vi "LDM111 main.vi"() -> ()   [LabVIEW 2012]
uses:
  <vilib>/DAQmx/read.llb/DAQmx Read (Analog 2D DBL NChan NSamp).vi
  <vilib>/DAQmx/write.llb/DAQmx Write (Digital 1D Bool 1Chan 1Samp).vi
  <vilib>/DAQmx/create/channels.llb/DAQmx Create Channel (CO-Pulse Generation-Frequency).vi
  <vilib>/DAQmx/configure/timing.llb/DAQmx Timing (Implicit).vi
  <vilib>/DAQmx/create/channels.llb/DAQmx Create Channel (AI-Voltage-Basic).vi
  <vilib>/DAQmx/configure/timing.llb/DAQmx Timing (Sample Clock).vi
  <vilib>/DAQmx/create/channels.llb/DAQmx Create Channel (DO-Digital Output).vi
  <vilib>/DAQmx/miscellaneous.llb/DAQmx Fill In Error Info.vi
  <resource>/objmgr/daqmx.rc
panel:
  in  "保存间隔时间":u64=1 min=1 step=1
  out "当前湿度":dbl min=0.0 format="%#.2f"
  in  "参数一致":bool
  in  "4-6参数设置":T1={"1-1"={TRUE, "占空比"=enum."100%", "运行时间"=99.0, "电压设置"=0.0}, "1-1 2"={FALSE, "占空比"=enum."0%", "运行时间"=0.0, "电压设置"=0.0}, "1-1 3"={FALSE, "占空比"=enum."0%", "运行时间"=0.0, "电压设置"=0.0}, "1-1 4"={FALSE, "占空比"=enum."0%", "运行时间"=0.0, "电压设置"=0.0}, "1-1 5"={FALSE, "占空比"=enum."0%", "运行时间"=0.0, "电压设置"=0.0}, "1-1 6"={FALSE, "占空比"=enum."0%", "运行时间"=0.0, "电压设置"=0.0}} {"1-1 6"."电压设置" min=0.0 format="%#.2f"; "1-1 6"."运行时间" min=0.0 format="%#.2f"; "1-1 5"."电压设置" min=0.0 format="%#.2f"; "1-1 5"."运行时间" min=0.0 format="%#.2f"; "1-1 4"."电压设置" min=0.0 format="%#.2f"; "1-1 4"."运行时间" min=0.0 format="%#.2f"; "1-1 3"."电压设置" min=0.0 format="%#.2f"; "1-1 3"."运行时间" min=0.0 format="%#.2f"; "1-1 2"."电压设置" min=0.0 format="%#.2f"; "1-1 2"."运行时间" min=0.0 format="%#.2f"; "1-1"."电压设置" min=0.0 format="%#.2f"; "1-1"."运行时间" min=0.0 format="%#.2f"}
  in  "1-3参数设置":T1={"1-1"={TRUE, "占空比"=enum."100%", "运行时间"=99.0, "电压设置"=13.5}, "1-1 2"={FALSE, "占空比"=enum."0%", "运行时间"=0.0, "电压设置"=0.0}, "1-1 3"={FALSE, "占空比"=enum."0%", "运行时间"=0.0, "电压设置"=0.0}, "1-1 4"={FALSE, "占空比"=enum."0%", "运行时间"=0.0, "电压设置"=0.0}, "1-1 5"={FALSE, "占空比"=enum."0%", "运行时间"=0.0, "电压设置"=0.0}, "1-1 6"={FALSE, "占空比"=enum."0%", "运行时间"=0.0, "电压设置"=0.0}} {"1-1 6"."电压设置" min=0.0 format="%#.2f"; "1-1 6"."运行时间" min=0.0 format="%#.2f"; "1-1 5"."电压设置" min=0.0 format="%#.2f"; "1-1 5"."运行时间" min=0.0 format="%#.2f"; "1-1 4"."电压设置" min=0.0 format="%#.2f"; "1-1 4"."运行时间" min=0.0 format="%#.2f"; "1-1 3"."电压设置" min=0.0 format="%#.2f"; "1-1 3"."运行时间" min=0.0 format="%#.2f"; "1-1 2"."电压设置" min=0.0 format="%#.2f"; "1-1 2"."运行时间" min=0.0 format="%#.2f"; "1-1"."电压设置" min=0.0 format="%#.2f"; "1-1"."运行时间" min=0.0 format="%#.2f"}
  in  "剩余时间":dbl min=0.0 format="%#.2f"
  in  "已运行时间":dbl min=0.0 format="%#.2f"
  in  "设定运行时间":dbl=999.0 min=0.0 format="%#.2f"
  in  "停止":bool
  in  "开始":bool
  out "当前温度":dbl min=0.0 format="%#.2f"
  out "工位6":T3={"输入电压"=0.0, "输入电流"=0.0, "输出电压"=0.0, "输出电流"=0.0, "工作效率"=0.0, "占空比"=0.0, "结果"=2.0} {"占空比" format="%#.2g"; "工作效率" format="%#.3f"; "输出电流" format="%#.1f"; "输出电压" format="%#.2f"; "输入电流" format="%#.1f"; "输入电压" format="%#.2f"}
  out "工位5":T3={"输入电压"=0.0, "输入电流"=0.0, "输出电压"=0.0, "输出电流"=0.0, "工作效率"=0.0, "占空比"=0.0, "结果"=2.0} {"占空比" format="%#.2g"; "工作效率" format="%#.3f"; "输出电流" format="%#.1f"; "输出电压" format="%#.2f"; "输入电流" format="%#.1f"; "输入电压" format="%#.2f"}
  out "工位4":T3={"输入电压"=0.0, "输入电流"=0.0, "输出电压"=0.0, "输出电流"=0.0, "工作效率"=0.0, "占空比"=0.0, "结果"=2.0} {"占空比" format="%#.2g"; "工作效率" format="%#.3f"; "输出电流" format="%#.1f"; "输出电压" format="%#.2f"; "输入电流" format="%#.1f"; "输入电压" format="%#.2f"}
  out "工位3":T3={"输入电压"=0.0, "输入电流"=0.0, "输出电压"=0.0, "输出电流"=0.0, "工作效率"=0.0, "占空比"=0.0, "结果"=2.0} {"占空比" format="%#.2g"; "工作效率" format="%#.3f"; "输出电流" format="%#.1f"; "输出电压" format="%#.2f"; "输入电流" format="%#.1f"; "输入电压" format="%#.2f"}
  out "工位2":T3={"输入电压"=0.0, "输入电流"=0.0, "输出电压"=0.0, "输出电流"=0.0, "工作效率"=0.0, "占空比"=0.0, "结果"=2.0} {"占空比" format="%#.2g"; "工作效率" format="%#.3f"; "输出电流" format="%#.1f"; "输出电压" format="%#.2f"; "输入电流" format="%#.1f"; "输入电压" format="%#.2f"}
  out "工位1":T3={"输入电压"=0.0, "输入电流"=0.0, "输出电压"=0.0, "输出电流"=0.0, "工作效率"=0.0, "占空比"=0.0, "结果"=2.0} {"占空比" format="%#.2g"; "工作效率" format="%#.3f"; "输出电流" format="%#.1f"; "输出电压" format="%#.2f"; "输入电流" format="%#.1f"; "输入电压" format="%#.2f"}
  # "LDM111"
  # "V"
  # "MA"
  # "V"
  # "MA"
  # "C"
  # "min"
  # "%"
  # "%"
  # "%"
  # "%"
  # "%"
  # "%"
  # "min"
  # "min"
  # "参数一致?"
  # "s"
  # "V"
  # "启用"
  # "min"
  # "V"
  # "启用"
  # "min"
  # "V"
  # "启用"
  # "min"
  # "启用"
  # "min"
  # "V"
  # "V"
  # "启用"
  # "min"
  # "启用"
  # "min"
  # "V"
  # "启用"
  # "V"
  # "min"
  # "启用"
  # "V"
  # "min"
  # "启用"
  # "V"
  # "min"
  # "启用"
  # "V"
  # "min"
  # "启用"
  # "V"
  # "min"
  # "启用"
  # "V"
  # "min"
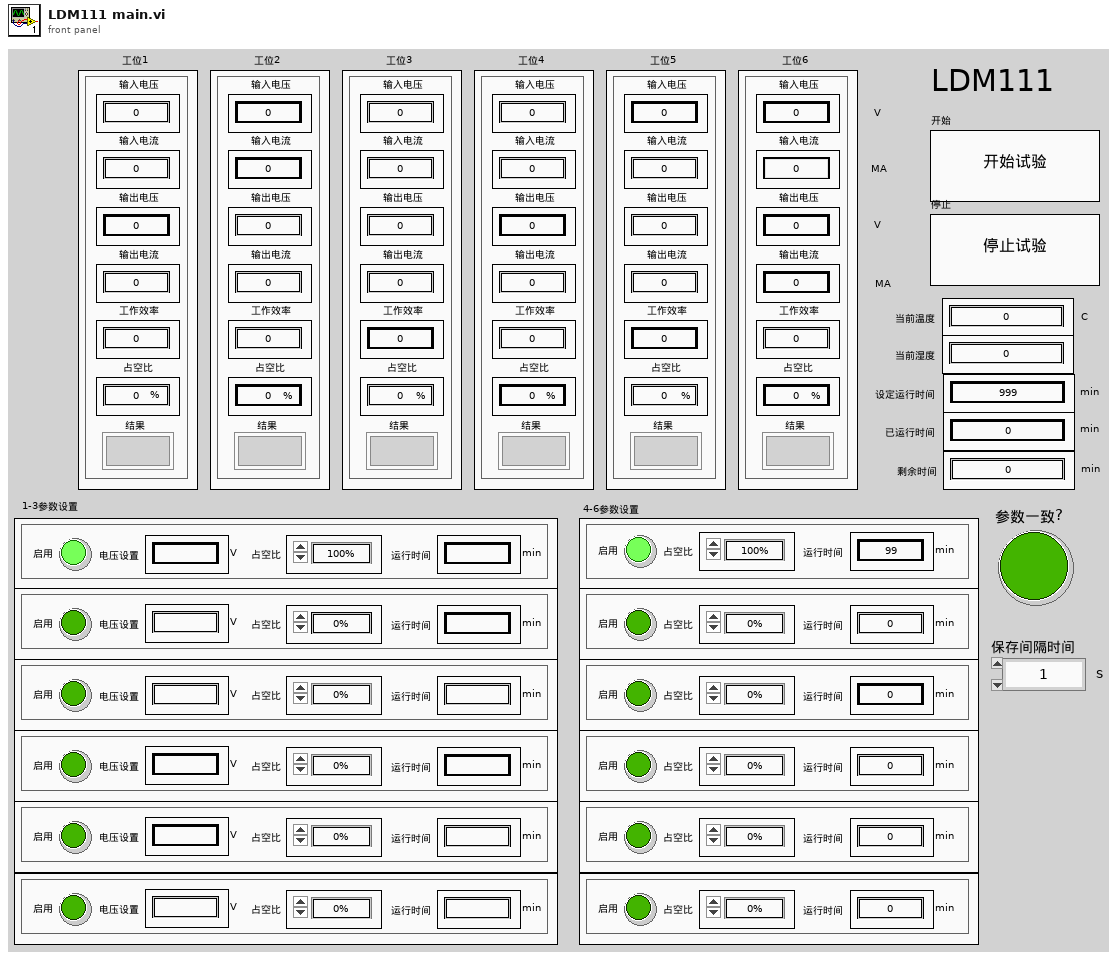
[diagram p1: front panel]
types:
  T1 = cluster{"1-1":cluster{bool, "占空比":enum16{"0%", "28%", "100%"}, "运行时间":dbl, "电压设置":dbl}, "1-1 2":cluster{bool, "占空比":enum16{"0%", "28%", "100%"}, "运行时间":dbl, "电压设置":dbl}, "1-1 3":cluster{bool, "占空比":enum16{"0%", "28%", "100%"}, "运行时间":dbl, "电压设置":dbl}, "1-1 4":cluster{bool, "占空比":enum16{"0%", "28%", "100%"}, "运行时间":dbl, "电压设置":dbl}, "1-1 5":cluster{bool, "占空比":enum16{"0%", "28%", "100%"}, "运行时间":dbl, "电压设置":dbl}, "1-1 6":cluster{bool, "占空比":enum16{"0%", "28%", "100%"}, "运行时间":dbl, "电压设置":dbl}}
  T2 = typedef "结果状态显示.ctl" = dbl
  T3 = cluster{"输入电压":dbl, "输入电流":dbl, "输出电压":dbl, "输出电流":dbl, "工作效率":dbl, "占空比":dbl, "结果":T2}
  T4 = typedef "控件 1.ctl" = enum16{"初始化", "空闲", "开始", "计时", "完成", "退出"}
  T5 = typedef "控件 3.ctl" = enum16{"初始化", "读取", "写入", "退出"}
  T6 = typedef "控件 2.ctl" = enum16{"创建事件", "产生事件", "销毁事件"}
  T7 = typedef "控件 4.ctl" = cluster{"工位1":refnum<vi>, "1-3参数设置":refnum<vi>, "总时间":u32, "NG？":bool, "循环次数":i32, "步骤次数":i32, "单个时间":u32, "完成?":bool, "路径":path, "1":i32, "2":i32, "3":i32, "4":i32, "AI":i32, "范围":i32, "保存间隔时间":u64}
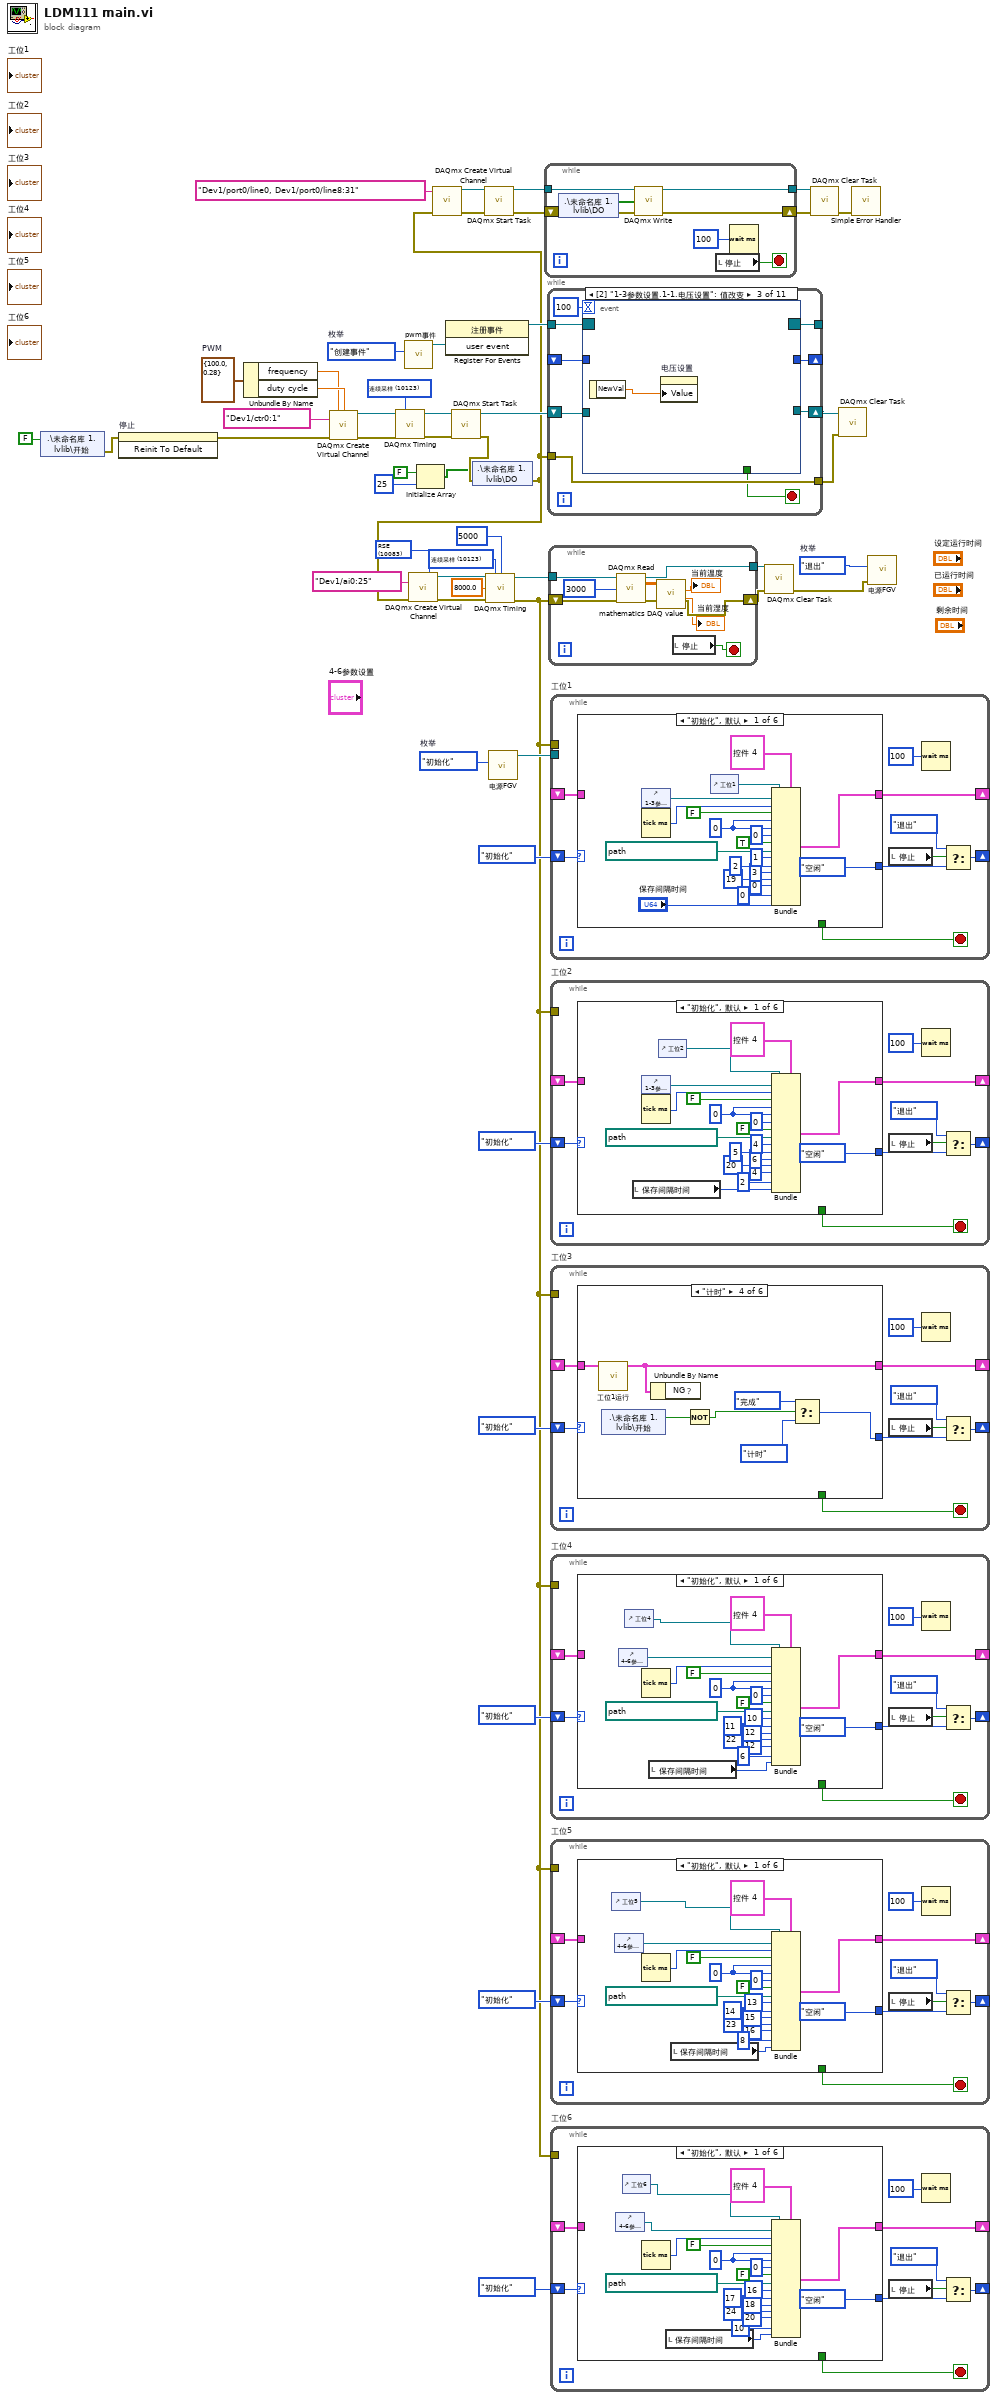
[diagram p0: block diagram]
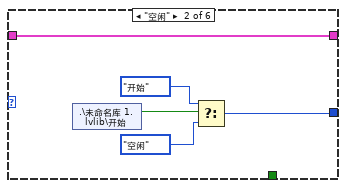
[diagram p2: hidden frame]
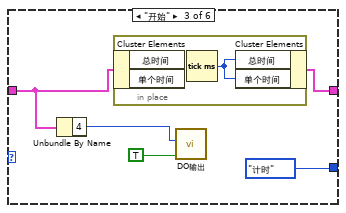
[diagram p3: hidden frame]
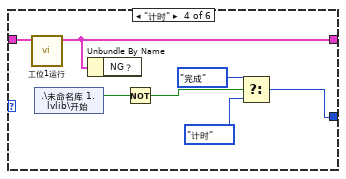
[diagram p4: hidden frame]
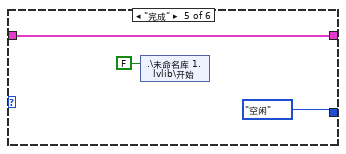
[diagram p5: hidden frame]
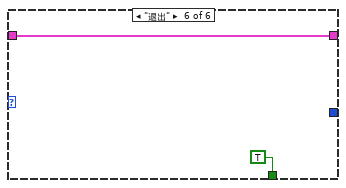
[diagram p6: hidden frame]
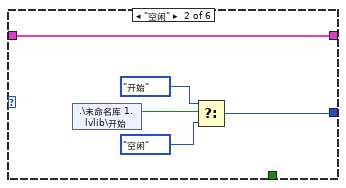
[diagram p7: hidden frame]
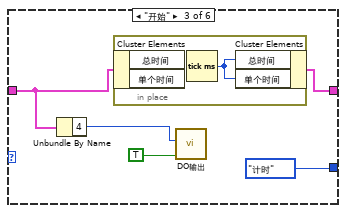
[diagram p8: hidden frame]
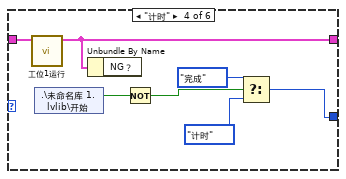
[diagram p9: hidden frame]
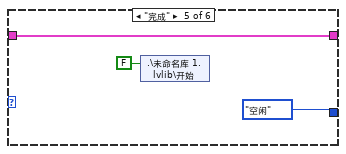
[diagram p10: hidden frame]
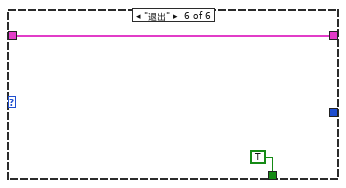
[diagram p11: hidden frame]
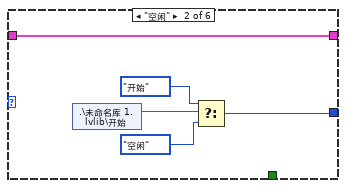
[diagram p12: hidden frame]
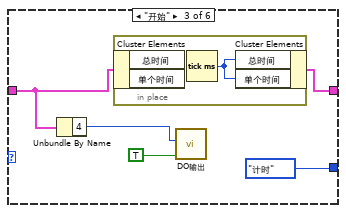
[diagram p13: hidden frame]
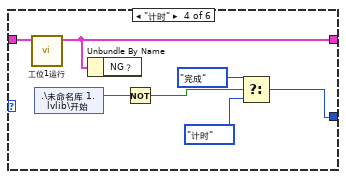
[diagram p14: hidden frame]
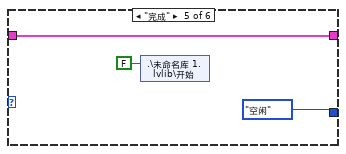
[diagram p15: hidden frame]
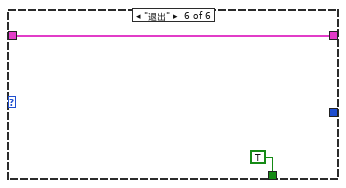
[diagram p16: hidden frame]
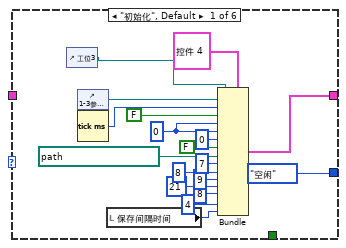
[diagram p17: hidden frame]
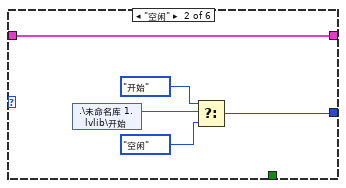
[diagram p18: hidden frame]
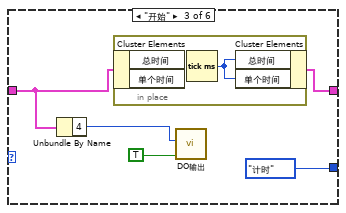
[diagram p19: hidden frame]
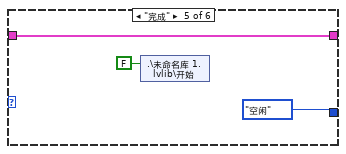
[diagram p20: hidden frame]
diagram:
  w8 = 控件_3."退出"  # 枚举
  w10 = 控件_3."初始化"  # 枚举
  w20 = 10083 items=["默认"=-1, "RSE"=10083, "NRSE"=10078, "差分"=10106, "伪差分"=12529] ("input terminal configuration")
  w22 = 10123 items=["有限采样"=10178, "连续采样"=10123, "硬件定时单点"=12522] ("sample mode")
  w34 = 10123 items=["有限采样"=10178, "连续采样"=10123, "硬件定时单点"=12522] ("sample mode")
  w37 = cluster{"frequency":dbl, "duty cycle":dbl} {"frequency"=100.0, "duty cycle"=0.28}  # PWM
  w44 = 控件_2."创建事件"  # 枚举
  n1 = shared-variable ".\\未命名库 1.lvlib\\开始"(FALSE ("开始")) -> (error out=w11:errorcluster)  [unwired: 1 in]
  n2 = invoke on="停止" class="Bool (严格)" method="Reinit To Default"(error in=w11) -> (error out=w26:errorcluster)  [unwired: 2 in, 2 out]
  n3 = Unbundle By Name(w37) -> ("frequency"=w39:dbl, "duty cycle"=w40:dbl)
  n4 = call-poly <vilib>:"DAQmx Create Virtual Channel.vi"("frequency"=w39, "duty cycle"=w40, "counter"=tag "Dev1/ctr0:1", "error in"=w26) -> ("task out"=w36:refnum<k21>, "error out"=w35:errorcluster)  [unwired: 10 in]
  n5 = call-poly <vilib>:"DAQmx Timing.vi"("task/channels in"=w36, "sample mode"=w34, "error in"=w35) -> ("task out"=w33:refnum<k21>, "error out"=w32:errorcluster)  [unwired: 11 in]
  n6 = call "pwm事件.vi"("枚举"=w44) -> ("user event"=w43:refnum<user-event>)  [unwired: 9 in, 1 out]
  n7 = Initialize Array(FALSE, 25 ("维数大小")) -> (w28:bool[])
  n8 = register-events(w43) -> (reference out=w42:refnum<event-registration>)  [unwired: 2 in, 1 out]
  n9 = call <vilib>:"DAQmx Start Task.vi"("task/channels in"=w33, "error in"=w32) -> ("task out"=w38:refnum<k21>, "error out"=w30:errorcluster)  [unwired: 12 in]
  n10 = shared-variable ".\\未命名库 1.lvlib\\DO"(w28, error in=w30) -> (error out=w17:errorcluster)
  n11 = call-poly <vilib>:"DAQmx Create Virtual Channel.vi"("input terminal configuration"=w20, "physical channels"=tag "Dev1/ai0:25", "error in"=w17) -> ("task out"=w25:refnum<k21>, "error out"=w24:errorcluster)  [unwired: 11 in]
  n12 = call-poly <vilib>:"DAQmx Create Virtual Channel.vi"("lines"=tag "Dev1/port0/line0, Dev1/port0/line8:31" ("Line(s)"), "error in"=w17) -> ("task out"=w45:refnum<k21>, "error out"=w46:errorcluster)  [unwired: 12 in]
  n13 = call <vilib>:"DAQmx Start Task.vi"("task/channels in"=w45, "error in"=w46) -> ("task out"=w52:refnum<k21>, "error out"=w51:errorcluster)  [unwired: 12 in]
  n14 = call-poly <vilib>:"DAQmx Timing.vi"("task/channels in"=w25, "sample mode"=w22, "samples per channel"=5000, "rate"=8000.0, "error in"=w24) -> ("task out"=w18:refnum<k21>, "error out"=w1:errorcluster)  [unwired: 9 in]
  n15 = call "电源FGV.vi"("枚举"=w10) -> ("VISA资源名称输出"=w9:refnum<visa-resource-name>)  [unwired: 9 in, 1 out]
  n16 = while {
    tunnel: w52 -> [w60]
    tunnel: [w59] -> w50
    shift-right: [w58] -> w49
    shift-left: w51 -> [w55]
    stop <- w53 stop-if-true
    n17 = shared-variable ".\\未命名库 1.lvlib\\DO"(error in=w55) -> (w56:bool[], error out=w54:errorcluster)
    n18 = call-poly <vilib>:"DAQmx Write.vi"("task/channels in"=w60, "data"=w56, "error in"=w54) -> ("task out"=w59:refnum<k21>, "error out"=w58:errorcluster)  [unwired: 10 in, 1 out]
    n19 = local read "停止"() -> (w53:bool)
    n20 = Wait (ms)(milliseconds to wait=u32 100 ("Loop Time (ms)")) -> ()  [unwired: 1 out]
  }
  n21 = while {
    tunnel: w42 -> [w69]
    tunnel: w17 -> [w64]
    tunnel: [w67] -> _
    shift-right: [w65] -> w41
    shift-left: w38 -> [w66]
    tunnel: [w64] -> w14
    shift-right: [w62] -> _
    shift-left: _ -> [w61]
    stop <- w63 stop-if-true
    n22 = event shown="[2] \"1-3参数设置.1-1.电压设置\": 值改变" {
      selector: w69 -> [_ _ _ _ _ _ _ _ _ _ _]
      dyn-events: [_ _ _ _ _ _ _ _ _ _ _] -> w67
      timeout: 100 -> [_ _ _ _ _ _ _ _ _ _ _]
      tunnel: w66 -> [w74 _ _ _ _ _ _ _ w84 _ _]
      tunnel: [w74 _ _ _ _ _ _ _ w83 _ _] -> w65
      tunnel: [_ _ _ _ _ _ _ _ _ _ TRUE ("开始")] -> w63
      tunnel: [w70 _ _ _ _ _ _ _ w82 w87 w92] -> w62
      tunnel: w61 -> [w70 _ _ _ _ _ _ _ w82 _ w92]
      event Timeout {
        n23 = event-data() -> ()  [unwired: 1 in, 2 out]
        n24 = control-ref of="剩余时间"() -> (w73:refnum<vi>)
        n25 = control-ref of="已运行时间"() -> (w72:refnum<vi>)
        n26 = control-ref of="设定运行时间"() -> (w71:refnum<vi>)
        n27 = call "总时间.vi"("已运行时间 2"=w72, "剩余时间 2"=w73, "设定运行时间 2"=w71, "millisecond timer value"=w70) -> ()  [unwired: 8 in]
      }
      event "参数一致": Value Change {
        n28 = event-data() -> ()  [unwired: 1 in, 5 out]
        n29 = local write "4-6参数设置"("1-3参数设置") -> ()
      }
      event "1-3参数设置.1-1.电压设置": Value Change {
        n30 = event-data() -> ("NewVal"=w76:dbl)  [unwired: 1 in]
        n31 = property on="电压设置" class="DigNum (严格)"("Value"=w76) -> ()  [unwired: 2 in, 2 out]
      }
      event "1-3参数设置.1-1 2.电压设置": Value Change {
        n32 = event-data() -> ("NewVal"=w77:dbl)  [unwired: 1 in]
        n33 = property on="电压设置" class="DigNum (严格)"("Value"=w77) -> ()  [unwired: 2 in, 2 out]
      }
      event "1-3参数设置.1-1 3.电压设置": Value Change {
        n34 = event-data() -> ("NewVal"=w78:dbl)  [unwired: 1 in]
        n35 = property on="电压设置" class="DigNum (严格)"("Value"=w78) -> ()  [unwired: 2 in, 2 out]
      }
      event "1-3参数设置.1-1 4.电压设置": Value Change {
        n36 = event-data() -> ("NewVal"=w79:dbl)  [unwired: 1 in]
        n37 = property on="电压设置" class="DigNum (严格)"("Value"=w79) -> ()  [unwired: 2 in, 2 out]
      }
      event "1-3参数设置.1-1 5.电压设置": Value Change {
        n38 = event-data() -> ("NewVal"=w80:dbl)  [unwired: 1 in]
        n39 = property on="电压设置" class="DigNum (严格)"("Value"=w80) -> ()  [unwired: 2 in, 2 out]
      }
      event "1-3参数设置.1-1 6.电压设置": Value Change {
        n40 = event-data() -> ("NewVal"=w81:dbl)  [unwired: 1 in]
        n41 = property on="电压设置" class="DigNum (严格)"("Value"=w81) -> ()  [unwired: 2 in, 2 out]
      }
      event User Event {
        n42 = event-data() -> ("frequency"=w86:dbl, "duty cycle"=w85:dbl)  [unwired: 1 in]
        n43 = property class="DAQmx通道"(reference=w84, "CO.Pulse.DutyCyc"=w85, "CO.Pulse.Freq"=w86) -> (reference out=w83:refnum<k21>)  [unwired: 1 in, 1 out]
      }
      event "开始": Value Change {
        n44 = event-data() -> ("NewVal"=w88:bool)  [unwired: 1 in, 1 out]
        n45 = shared-variable ".\\未命名库 1.lvlib\\开始"(w88) -> ()  [unwired: 1 in, 1 out]
        n46 = Tick Count (ms)() -> (millisecond timer value=w87:u32)
      }
      event "停止": Value Change {
        n47 = event-data() -> ()  [unwired: 1 in, 1 out]
        n48 = Initialize Array(FALSE, 25 ("维数大小")) -> (w89:bool[])
        n49 = shared-variable ".\\未命名库 1.lvlib\\DO"(w89) -> ()  [unwired: 1 in, 1 out]
        n50 = shared-variable ".\\未命名库 1.lvlib\\开始"(FALSE ("开始")) -> ()  [unwired: 1 in, 1 out]
      }
    }
  }
  n51 = while {
    tunnel: w18 -> [w102]
    shift-right: [w98] -> w15
    shift-left: w1 -> [w101]
    tunnel: [w100] -> w16
    stop <- w97 stop-if-true
    n52 = call-poly <vilib>:"DAQmx Read.vi"("task/channels in"=w102, "number of samples per channel"=3000, "error in"=w101) -> ("task out"=w100:refnum<k21>, "data"=w99:dbl[][], "error out"=w98:errorcluster)  [unwired: 10 in]
    n53 = call "mathematics DAQ value.vi"("Array"=w99) -> ("湿度?"=→"当前湿度":dbl, "温度?"=→"当前温度":dbl)  [unwired: 4 in, 1 out]
    n54 = local read "停止"() -> (w97:bool)
  }
  n55 = while "工位1" {
    shift-right: [w109] -> _
    shift-left: 控件_1."初始化" ("枚举") -> [w112]
    shift-right: [w108] -> _
    shift-left: _ -> [w107]
    tunnel: w1 -> [_]
    tunnel: w9 -> [_]
    stop <- w105 stop-if-true
    n56 = case shown="\"初始化\", 默认" w112 {
      tunnel: [w128 w131 w139 w147 w151 w153] -> w108
      tunnel: w107 -> [_ w131 w137 w148 w151 w153]
      tunnel: [控件_1."空闲" ("枚举") w132 控件_1."计时" ("枚举") w144 控件_1."空闲" ("枚举") _] -> w106
      tunnel: [_ _ _ _ _ TRUE] -> w105
      frame "初始化", Default {
        w125 = 0 ("步骤次数")
        n57 = control-ref of="1-3参数设置"() -> (w129:refnum<vi>)
        n58 = Tick Count (ms)() -> (millisecond timer value=w127:u32)
        n59 = control-ref of="工位1"() -> (w130:refnum<vi>)
        n60 = Bundle(cluster=T7 {"工位1"=refnum, "1-3参数设置"=refnum, "总时间"=0, "NG？"=FALSE, "循环次数"=0, "步骤次数"=0, "单个时间"=0, "完成?"=FALSE, "路径"=path "e:/LDM数据/工位一", "1"=19, "2"=19, "3"=19, "4"=19, "AI"=24, "范围"=24, "保存间隔时间"=0} ("簇 2"), "工位1"=w130, "1-3参数设置"=w129, "总时间"=w127, "NG？"=FALSE, "循环次数"=w125, "步骤次数"=w125, "单个时间"=u32 0, "完成?"=TRUE, "路径"=path "e:/LDM数据/工位一", "1"=1, "2"=2 ("1"), "3"=3 ("1"), "4"=19 ("1"), "AI"=0 ("1"), "范围"=0 ("1"), "保存间隔时间"="保存间隔时间") -> (w128:T7)
      }
      frame "空闲" {
        n61 = shared-variable ".\\未命名库 1.lvlib\\开始"() -> (w135:bool)  [unwired: 1 in, 1 out]
        n62 = Select(t=控件_1."开始" ("枚举"), s=w135, f=控件_1."空闲" ("枚举")) -> (s? t:f=w132:T4)
      }
      frame "开始" {
        n63 = Unbundle By Name(w137) -> ("4"=w136:i32)
        n64 = in-place {
          n65 = in-place-cluster #1(w137) -> ()  [unwired: 2 out]
          n66 = Tick Count (ms)() -> (millisecond timer value=w141:u32)
          n67 = in-place-cluster #1("总时间"=w141, "单个时间"=w141) -> (w139:T7)
        }
        n68 = call "DO输出.vi"("TF"=TRUE, "序号"=w136) -> ()  [unwired: 9 in, 1 out]
      }
      frame "计时" {
        n69 = call "工位1运行.vi"("簇"=w148) -> ("簇 2"=w147:T7)  [unwired: 10 in]
        n70 = shared-variable ".\\未命名库 1.lvlib\\开始"() -> (w143:bool)  [unwired: 1 in, 1 out]
        n71 = Unbundle By Name(w147) -> ()  [unwired: 1 out]
        n72 = Not(x=w143) -> (.not. x?=w142:bool)
        n73 = Select(t=控件_1."完成" ("枚举"), s=w142, f=控件_1."计时" ("枚举")) -> (s? t:f=w144:T4)
      }
      frame "完成" {
        n74 = shared-variable ".\\未命名库 1.lvlib\\开始"(FALSE ("开始")) -> ()  [unwired: 1 in, 1 out]
      }
      frame "退出" {
      }
    }
    n75 = local read "停止"() -> (w111:bool)
    n76 = Wait (ms)(milliseconds to wait=u32 100 ("等待时间（毫秒）")) -> ()  [unwired: 1 out]
    n77 = Select(t=控件_1."退出" ("枚举"), s=w111, f=w106) -> (s? t:f=w109:T4)
  }
  n78 = while "工位2" {
    shift-right: [w159] -> _
    shift-left: 控件_1."初始化" ("枚举") -> [w162]
    shift-right: [w158] -> _
    shift-left: _ -> [w157]
    tunnel: w1 -> [_]
    stop <- w155 stop-if-true
    n79 = case shown="\"初始化\", 默认" w162 {
      tunnel: [w179 w181 w189 w197 w201 w203] -> w158
      tunnel: w157 -> [_ w181 w187 w198 w201 w203]
      tunnel: [控件_1."空闲" ("枚举") w182 控件_1."计时" ("枚举") w194 控件_1."空闲" ("枚举") _] -> w156
      tunnel: [_ _ _ _ _ TRUE] -> w155
      frame "初始化", Default {
        w176 = 0 ("步骤次数")
        n80 = local read "保存间隔时间"() -> (w163:u64)
        n81 = control-ref of="1-3参数设置"() -> (w180:refnum<vi>)
        n82 = Tick Count (ms)() -> (millisecond timer value=w178:u32)
        n83 = control-ref of="工位2"() -> (w165:refnum<vi>)
        n84 = Bundle(cluster=T7 {"工位1"=refnum, "1-3参数设置"=refnum, "总时间"=0, "NG？"=FALSE, "循环次数"=0, "步骤次数"=0, "单个时间"=0, "完成?"=FALSE, "路径"=path "e:/LDM数据/工位一", "1"=19, "2"=19, "3"=19, "4"=19, "AI"=24, "范围"=24, "保存间隔时间"=0} ("簇 2"), "工位1"=w165, "1-3参数设置"=w180, "总时间"=w178, "NG？"=FALSE, "循环次数"=w176, "步骤次数"=w176, "单个时间"=u32 0, "完成?"=FALSE, "路径"=path "e:/LDM数据/工位二", "1"=4, "2"=5 ("1"), "3"=6 ("1"), "4"=20 ("1"), "AI"=4 ("1"), "范围"=2 ("1"), "保存间隔时间"=w163) -> (w179:T7)
      }
      frame "空闲" {
        n85 = shared-variable ".\\未命名库 1.lvlib\\开始"() -> (w185:bool)  [unwired: 1 in, 1 out]
        n86 = Select(t=控件_1."开始" ("枚举"), s=w185, f=控件_1."空闲" ("枚举")) -> (s? t:f=w182:T4)
      }
      frame "开始" {
        n87 = Unbundle By Name(w187) -> ("4"=w186:i32)
        n88 = in-place {
          n89 = in-place-cluster #2(w187) -> ()  [unwired: 2 out]
          n90 = Tick Count (ms)() -> (millisecond timer value=w191:u32)
          n91 = in-place-cluster #2("总时间"=w191, "单个时间"=w191) -> (w189:T7)
        }
        n92 = call "DO输出.vi"("TF"=TRUE, "序号"=w186) -> ()  [unwired: 9 in, 1 out]
      }
      frame "计时" {
        n93 = call "工位1运行.vi"("簇"=w198) -> ("簇 2"=w197:T7)  [unwired: 10 in]
        n94 = shared-variable ".\\未命名库 1.lvlib\\开始"() -> (w193:bool)  [unwired: 1 in, 1 out]
        n95 = Unbundle By Name(w197) -> ()  [unwired: 1 out]
        n96 = Not(x=w193) -> (.not. x?=w192:bool)
        n97 = Select(t=控件_1."完成" ("枚举"), s=w192, f=控件_1."计时" ("枚举")) -> (s? t:f=w194:T4)
      }
      frame "完成" {
        n98 = shared-variable ".\\未命名库 1.lvlib\\开始"(FALSE ("开始")) -> ()  [unwired: 1 in, 1 out]
      }
      frame "退出" {
      }
    }
    n99 = local read "停止"() -> (w161:bool)
    n100 = Wait (ms)(milliseconds to wait=u32 100 ("等待时间（毫秒）")) -> ()  [unwired: 1 out]
    n101 = Select(t=控件_1."退出" ("枚举"), s=w161, f=w156) -> (s? t:f=w159:T4)
  }
  n102 = while "工位3" {
    shift-right: [w209] -> _
    shift-left: 控件_1."初始化" ("枚举") -> [w212]
    shift-right: [w208] -> _
    shift-left: _ -> [w207]
    tunnel: w1 -> [_]
    stop <- w205 stop-if-true
    n103 = case shown="\"计时\"" w212 {
      tunnel: [w229 w231 w239 w247 w251 w253] -> w208
      tunnel: w207 -> [_ w231 w237 w248 w251 w253]
      tunnel: [控件_1."空闲" ("枚举") w232 控件_1."计时" ("枚举") w244 控件_1."空闲" ("枚举") _] -> w206
      tunnel: [_ _ _ _ _ TRUE] -> w205
      frame "初始化", Default {
        w226 = 0 ("步骤次数")
        n104 = control-ref of="工位3"() -> (w214:refnum<vi>)
        n105 = control-ref of="1-3参数设置"() -> (w230:refnum<vi>)
        n106 = Tick Count (ms)() -> (millisecond timer value=w228:u32)
        n107 = local read "保存间隔时间"() -> (w213:u64)
        n108 = Bundle(cluster=T7 {"工位1"=refnum, "1-3参数设置"=refnum, "总时间"=0, "NG？"=FALSE, "循环次数"=0, "步骤次数"=0, "单个时间"=0, "完成?"=FALSE, "路径"=path "e:/LDM数据/工位一", "1"=19, "2"=19, "3"=19, "4"=19, "AI"=24, "范围"=24, "保存间隔时间"=0} ("簇 2"), "工位1"=w214, "1-3参数设置"=w230, "总时间"=w228, "NG？"=FALSE, "循环次数"=w226, "步骤次数"=w226, "单个时间"=u32 0, "完成?"=FALSE, "路径"=path "e:/LDM数据/工位三", "1"=7, "2"=8 ("1"), "3"=9 ("1"), "4"=21 ("1"), "AI"=8 ("1"), "范围"=4 ("1"), "保存间隔时间"=w213) -> (w229:T7)
      }
      frame "空闲" {
        n109 = shared-variable ".\\未命名库 1.lvlib\\开始"() -> (w235:bool)  [unwired: 1 in, 1 out]
        n110 = Select(t=控件_1."开始" ("枚举"), s=w235, f=控件_1."空闲" ("枚举")) -> (s? t:f=w232:T4)
      }
      frame "开始" {
        n111 = Unbundle By Name(w237) -> ("4"=w236:i32)
        n112 = in-place {
          n113 = in-place-cluster #3(w237) -> ()  [unwired: 2 out]
          n114 = Tick Count (ms)() -> (millisecond timer value=w241:u32)
          n115 = in-place-cluster #3("总时间"=w241, "单个时间"=w241) -> (w239:T7)
        }
        n116 = call "DO输出.vi"("TF"=TRUE, "序号"=w236) -> ()  [unwired: 9 in, 1 out]
      }
      frame "计时" {
        n117 = call "工位1运行.vi"("簇"=w248) -> ("簇 2"=w247:T7)  [unwired: 10 in]
        n118 = shared-variable ".\\未命名库 1.lvlib\\开始"() -> (w243:bool)  [unwired: 1 in, 1 out]
        n119 = Unbundle By Name(w247) -> ()  [unwired: 1 out]
        n120 = Not(x=w243) -> (.not. x?=w242:bool)
        n121 = Select(t=控件_1."完成" ("枚举"), s=w242, f=控件_1."计时" ("枚举")) -> (s? t:f=w244:T4)
      }
      frame "完成" {
        n122 = shared-variable ".\\未命名库 1.lvlib\\开始"(FALSE ("开始")) -> ()  [unwired: 1 in, 1 out]
      }
      frame "退出" {
      }
    }
    n123 = local read "停止"() -> (w211:bool)
    n124 = Wait (ms)(milliseconds to wait=u32 100 ("等待时间（毫秒）")) -> ()  [unwired: 1 out]
    n125 = Select(t=控件_1."退出" ("枚举"), s=w211, f=w206) -> (s? t:f=w209:T4)
  }
  n126 = while "工位4" {
    shift-right: [w259] -> _
    shift-left: 控件_1."初始化" ("枚举") -> [w262]
    shift-right: [w258] -> _
    shift-left: _ -> [w257]
    tunnel: w1 -> [_]
    stop <- w255 stop-if-true
    n127 = case shown="\"初始化\", 默认" w262 {
      tunnel: [w280 w281 w289 w297 w301 w303] -> w258
      tunnel: w257 -> [_ w281 w287 w298 w301 w303]
      tunnel: [控件_1."空闲" ("枚举") w282 控件_1."计时" ("枚举") w294 控件_1."空闲" ("枚举") _] -> w256
      tunnel: [_ _ _ _ _ TRUE] -> w255
      frame "初始化", Default {
        w277 = 0 ("步骤次数")
        n128 = control-ref of="4-6参数设置"() -> (w265:refnum<vi>)
        n129 = control-ref of="工位4"() -> (w264:refnum<vi>)
        n130 = Tick Count (ms)() -> (millisecond timer value=w279:u32)
        n131 = local read "保存间隔时间"() -> (w263:u64)
        n132 = Bundle(cluster=T7 {"工位1"=refnum, "1-3参数设置"=refnum, "总时间"=0, "NG？"=FALSE, "循环次数"=0, "步骤次数"=0, "单个时间"=0, "完成?"=FALSE, "路径"=path "e:/LDM数据/工位一", "1"=19, "2"=19, "3"=19, "4"=19, "AI"=24, "范围"=24, "保存间隔时间"=0} ("簇 2"), "工位1"=w264, "1-3参数设置"=w265, "总时间"=w279, "NG？"=FALSE, "循环次数"=w277, "步骤次数"=w277, "单个时间"=u32 0, "完成?"=FALSE, "路径"=path "e:/LDM数据/工位四", "1"=10, "2"=11 ("1"), "3"=12 ("1"), "4"=22 ("1"), "AI"=12 ("1"), "范围"=6 ("1"), "保存间隔时间"=w263) -> (w280:T7)
      }
      frame "空闲" {
        n133 = shared-variable ".\\未命名库 1.lvlib\\开始"() -> (w285:bool)  [unwired: 1 in, 1 out]
        n134 = Select(t=控件_1."开始" ("枚举"), s=w285, f=控件_1."空闲" ("枚举")) -> (s? t:f=w282:T4)
      }
      frame "开始" {
        n135 = Unbundle By Name(w287) -> ("4"=w286:i32)
        n136 = in-place {
          n137 = in-place-cluster #4(w287) -> ()  [unwired: 2 out]
          n138 = Tick Count (ms)() -> (millisecond timer value=w291:u32)
          n139 = in-place-cluster #4("总时间"=w291, "单个时间"=w291) -> (w289:T7)
        }
        n140 = call "DO输出.vi"("TF"=TRUE, "序号"=w286) -> ()  [unwired: 9 in, 1 out]
      }
      frame "计时" {
        n141 = call "工位1运行.vi"("簇"=w298) -> ("簇 2"=w297:T7)  [unwired: 10 in]
        n142 = shared-variable ".\\未命名库 1.lvlib\\开始"() -> (w293:bool)  [unwired: 1 in, 1 out]
        n143 = Unbundle By Name(w297) -> ()  [unwired: 1 out]
        n144 = Not(x=w293) -> (.not. x?=w292:bool)
        n145 = Select(t=控件_1."完成" ("枚举"), s=w292, f=控件_1."计时" ("枚举")) -> (s? t:f=w294:T4)
      }
      frame "完成" {
        n146 = shared-variable ".\\未命名库 1.lvlib\\开始"(FALSE ("开始")) -> ()  [unwired: 1 in, 1 out]
      }
      frame "退出" {
      }
    }
    n147 = local read "停止"() -> (w261:bool)
    n148 = Wait (ms)(milliseconds to wait=u32 100 ("等待时间（毫秒）")) -> ()  [unwired: 1 out]
    n149 = Select(t=控件_1."退出" ("枚举"), s=w261, f=w256) -> (s? t:f=w259:T4)
  }
  n150 = while "工位5" {
    shift-right: [w309] -> _
    shift-left: 控件_1."初始化" ("枚举") -> [w312]
    shift-right: [w308] -> _
    shift-left: _ -> [w307]
    tunnel: w1 -> [_]
    stop <- w305 stop-if-true
    n151 = case shown="\"初始化\", 默认" w312 {
      tunnel: [w330 w331 w339 w347 w351 w353] -> w308
      tunnel: w307 -> [_ w331 w337 w348 w351 w353]
      tunnel: [控件_1."空闲" ("枚举") w332 控件_1."计时" ("枚举") w344 控件_1."空闲" ("枚举") _] -> w306
      tunnel: [_ _ _ _ _ TRUE] -> w305
      frame "初始化", Default {
        w327 = 0 ("步骤次数")
        n152 = control-ref of="工位5"() -> (w314:refnum<vi>)
        n153 = control-ref of="4-6参数设置"() -> (w315:refnum<vi>)
        n154 = Tick Count (ms)() -> (millisecond timer value=w329:u32)
        n155 = local read "保存间隔时间"() -> (w313:u64)
        n156 = Bundle(cluster=T7 {"工位1"=refnum, "1-3参数设置"=refnum, "总时间"=0, "NG？"=FALSE, "循环次数"=0, "步骤次数"=0, "单个时间"=0, "完成?"=FALSE, "路径"=path "e:/LDM数据/工位一", "1"=19, "2"=19, "3"=19, "4"=19, "AI"=24, "范围"=24, "保存间隔时间"=0} ("簇 2"), "工位1"=w314, "1-3参数设置"=w315, "总时间"=w329, "NG？"=FALSE, "循环次数"=w327, "步骤次数"=w327, "单个时间"=u32 0, "完成?"=FALSE, "路径"=path "e:/LDM数据/工位五", "1"=13, "2"=14 ("1"), "3"=15 ("1"), "4"=23 ("1"), "AI"=16 ("1"), "范围"=8 ("1"), "保存间隔时间"=w313) -> (w330:T7)
      }
      frame "空闲" {
        n157 = shared-variable ".\\未命名库 1.lvlib\\开始"() -> (w335:bool)  [unwired: 1 in, 1 out]
        n158 = Select(t=控件_1."开始" ("枚举"), s=w335, f=控件_1."空闲" ("枚举")) -> (s? t:f=w332:T4)
      }
      frame "开始" {
        n159 = Unbundle By Name(w337) -> ("4"=w336:i32)
        n160 = in-place {
          n161 = in-place-cluster #5(w337) -> ()  [unwired: 2 out]
          n162 = Tick Count (ms)() -> (millisecond timer value=w341:u32)
          n163 = in-place-cluster #5("总时间"=w341, "单个时间"=w341) -> (w339:T7)
        }
        n164 = call "DO输出.vi"("TF"=TRUE, "序号"=w336) -> ()  [unwired: 9 in, 1 out]
      }
      frame "计时" {
        n165 = call "工位1运行.vi"("簇"=w348) -> ("簇 2"=w347:T7)  [unwired: 10 in]
        n166 = shared-variable ".\\未命名库 1.lvlib\\开始"() -> (w343:bool)  [unwired: 1 in, 1 out]
        n167 = Unbundle By Name(w347) -> ()  [unwired: 1 out]
        n168 = Not(x=w343) -> (.not. x?=w342:bool)
        n169 = Select(t=控件_1."完成" ("枚举"), s=w342, f=控件_1."计时" ("枚举")) -> (s? t:f=w344:T4)
      }
      frame "完成" {
        n170 = shared-variable ".\\未命名库 1.lvlib\\开始"(FALSE ("开始")) -> ()  [unwired: 1 in, 1 out]
      }
      frame "退出" {
      }
    }
    n171 = local read "停止"() -> (w311:bool)
    n172 = Wait (ms)(milliseconds to wait=u32 100 ("等待时间（毫秒）")) -> ()  [unwired: 1 out]
    n173 = Select(t=控件_1."退出" ("枚举"), s=w311, f=w306) -> (s? t:f=w309:T4)
  }
  n174 = while "工位6" {
    shift-right: [w359] -> _
    shift-left: 控件_1."初始化" ("枚举") -> [w362]
    shift-right: [w358] -> _
    shift-left: _ -> [w357]
    tunnel: w1 -> [_]
    stop <- w355 stop-if-true
    n175 = case shown="\"初始化\", 默认" w362 {
      tunnel: [w380 w381 w389 w397 w401 w403] -> w358
      tunnel: w357 -> [_ w381 w387 w398 w401 w403]
      tunnel: [控件_1."空闲" ("枚举") w382 控件_1."计时" ("枚举") w394 控件_1."空闲" ("枚举") _] -> w356
      tunnel: [_ _ _ _ _ TRUE] -> w355
      frame "初始化", Default {
        w377 = 0 ("步骤次数")
        n176 = control-ref of="4-6参数设置"() -> (w364:refnum<vi>)
        n177 = control-ref of="工位6"() -> (w365:refnum<vi>)
        n178 = Tick Count (ms)() -> (millisecond timer value=w379:u32)
        n179 = local read "保存间隔时间"() -> (w363:u64)
        n180 = Bundle(cluster=T7 {"工位1"=refnum, "1-3参数设置"=refnum, "总时间"=0, "NG？"=FALSE, "循环次数"=0, "步骤次数"=0, "单个时间"=0, "完成?"=FALSE, "路径"=path "e:/LDM数据/工位一", "1"=19, "2"=19, "3"=19, "4"=19, "AI"=24, "范围"=24, "保存间隔时间"=0} ("簇 2"), "工位1"=w365, "1-3参数设置"=w364, "总时间"=w379, "NG？"=FALSE, "循环次数"=w377, "步骤次数"=w377, "单个时间"=u32 0, "完成?"=FALSE, "路径"=path "e:/LDM数据/工位六", "1"=16, "2"=17 ("1"), "3"=18 ("1"), "4"=24 ("1"), "AI"=20 ("1"), "范围"=10 ("1"), "保存间隔时间"=w363) -> (w380:T7)
      }
      frame "空闲" {
        n181 = shared-variable ".\\未命名库 1.lvlib\\开始"() -> (w385:bool)  [unwired: 1 in, 1 out]
        n182 = Select(t=控件_1."开始" ("枚举"), s=w385, f=控件_1."空闲" ("枚举")) -> (s? t:f=w382:T4)
      }
      frame "开始" {
        n183 = Unbundle By Name(w387) -> ("4"=w386:i32)
        n184 = in-place {
          n185 = in-place-cluster #6(w387) -> ()  [unwired: 2 out]
          n186 = Tick Count (ms)() -> (millisecond timer value=w391:u32)
          n187 = in-place-cluster #6("总时间"=w391, "单个时间"=w391) -> (w389:T7)
        }
        n188 = call "DO输出.vi"("TF"=TRUE, "序号"=w386) -> ()  [unwired: 9 in, 1 out]
      }
      frame "计时" {
        n189 = call "工位1运行.vi"("簇"=w398) -> ("簇 2"=w397:T7)  [unwired: 10 in]
        n190 = shared-variable ".\\未命名库 1.lvlib\\开始"() -> (w393:bool)  [unwired: 1 in, 1 out]
        n191 = Unbundle By Name(w397) -> ()  [unwired: 1 out]
        n192 = Not(x=w393) -> (.not. x?=w392:bool)
        n193 = Select(t=控件_1."完成" ("枚举"), s=w392, f=控件_1."计时" ("枚举")) -> (s? t:f=w394:T4)
      }
      frame "完成" {
        n194 = shared-variable ".\\未命名库 1.lvlib\\开始"(FALSE ("开始")) -> ()  [unwired: 1 in, 1 out]
      }
      frame "退出" {
      }
    }
    n195 = local read "停止"() -> (w361:bool)
    n196 = Wait (ms)(milliseconds to wait=u32 100 ("等待时间（毫秒）")) -> ()  [unwired: 1 out]
    n197 = Select(t=控件_1."退出" ("枚举"), s=w361, f=w356) -> (s? t:f=w359:T4)
  }
  n198 = call <vilib>:"DAQmx Clear Task.vi"("task in"=w16, "error in"=w15) -> ("error out"=w7:errorcluster)  [unwired: 13 in]
  n199 = call <vilib>:"DAQmx Clear Task.vi"("task in"=w50, "error in"=w49) -> ("error out"=w48:errorcluster)  [unwired: 13 in]
  n200 = call <vilib>:"DAQmx Clear Task.vi"("task in"=w41, "error in"=w14) -> ()  [unwired: 13 in, 1 out]
  n201 = call <vilib>:"Simple Error Handler.vi"("error in (no error)"=w48) -> ()  [unwired: 4 in, 5 out]
  n202 = call "电源FGV.vi"("error in (no error)"=w7, "枚举"=w8) -> ()  [unwired: 8 in, 2 out]
